vi "Set Panel Update State.vi"(7 "Defer?":bool, 8 "error in (no error)":errorcluster, 11 "MenuButton Event Handler in":refnum<class "MenuButton Event Handler.lvclass">) -> (0 "error out":errorcluster, 3 "MenuButton Event Handler out":refnum<class "MenuButton Event Handler.lvclass">)   [LabVIEW 2017, in "MenuButtons.lvlib" / "MenuButton Event Handler.lvclass"]
uses:
  MenuButton Event Handler.lvclass
  MenuButton Event Handler.lvclass/MenuButton Event Handler.ctl
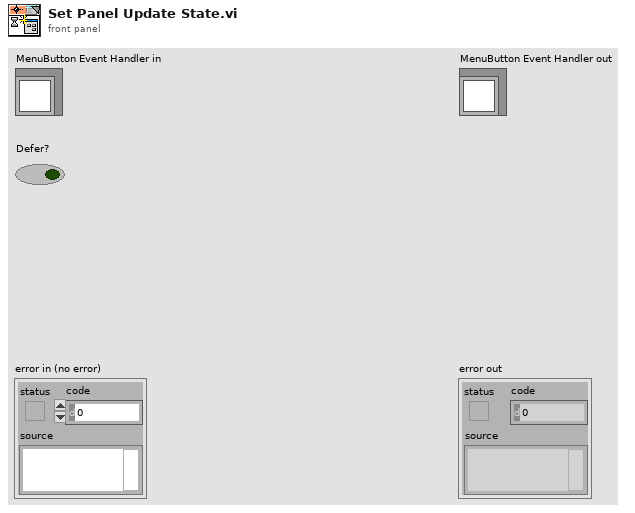
[diagram p1: front panel]
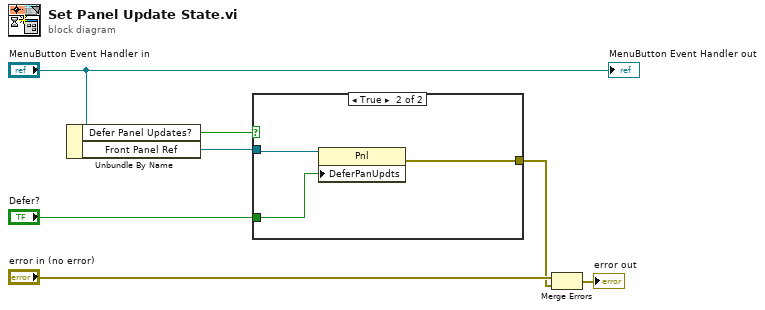
[diagram p0: block diagram]
diagram:
  n1 = Unbundle By Name("MenuButton Event Handler in") -> ("Defer Panel Updates?"=w5:bool, "Front Panel Ref"=w4:refnum<vi>)
  n2 = case shown="True" w5 {
    tunnel: w4 -> [_ w10]
    tunnel: "Defer?" -> [_ w9]
    tunnel: [_ w8] -> w1
    frame False {
    }
    frame True {
      n3 = property class="Pnl"(reference=w10, "DeferPanUpdts"=w9) -> (error out=w8:errorcluster)  [unwired: 1 in, 1 out]
    }
  }
  n4 = Merge Errors("error in (no error)", w1) -> (→"error out":errorcluster)
  "MenuButton Event Handler out" <- "MenuButton Event Handler in"
